vi "DroneTcpConnectionMovement.vi"() -> ()   [LabVIEW 2017]
uses:
  <vilib>/userdefined/High Color/IMAQdx.ctl
  <vilib>/vision/driver/IMAQdx.llb/IMAQdx Camera Control Mode.ctl
  <vilib>/vision/driver/NI_Vision_Acquisition_Software.lvlib
panel:
  in  "stop 3":bool
  in  "Snap":bool
  out "x":dbl
  out "created path":path
  in  "error in":errorcluster
  in  "Image Type":T1 items=["Grayscale (U8)", "Grayscale (I16)", "Grayscale (SGL)", "Complex (CSG)", "RGB (U32)", "HSL (U32)", "RGB (U64)", "Grayscale (U16)"]
  in  "Session In":T2
  in  "stop 2":bool
  out "Image":T3(plugin-control)
  out "unsigned byte array":u8[](array[numeric])
  out "Python server reply":string
  in  "stop":bool
  out "Control cluster":T4 {"Roll" scale=-1.0..1.0; "Pitch" scale=-1.0..1.0; "Vertical Speed" scale=-1.0..1.0; "Yaw Speed" scale=-1.0..1.0}
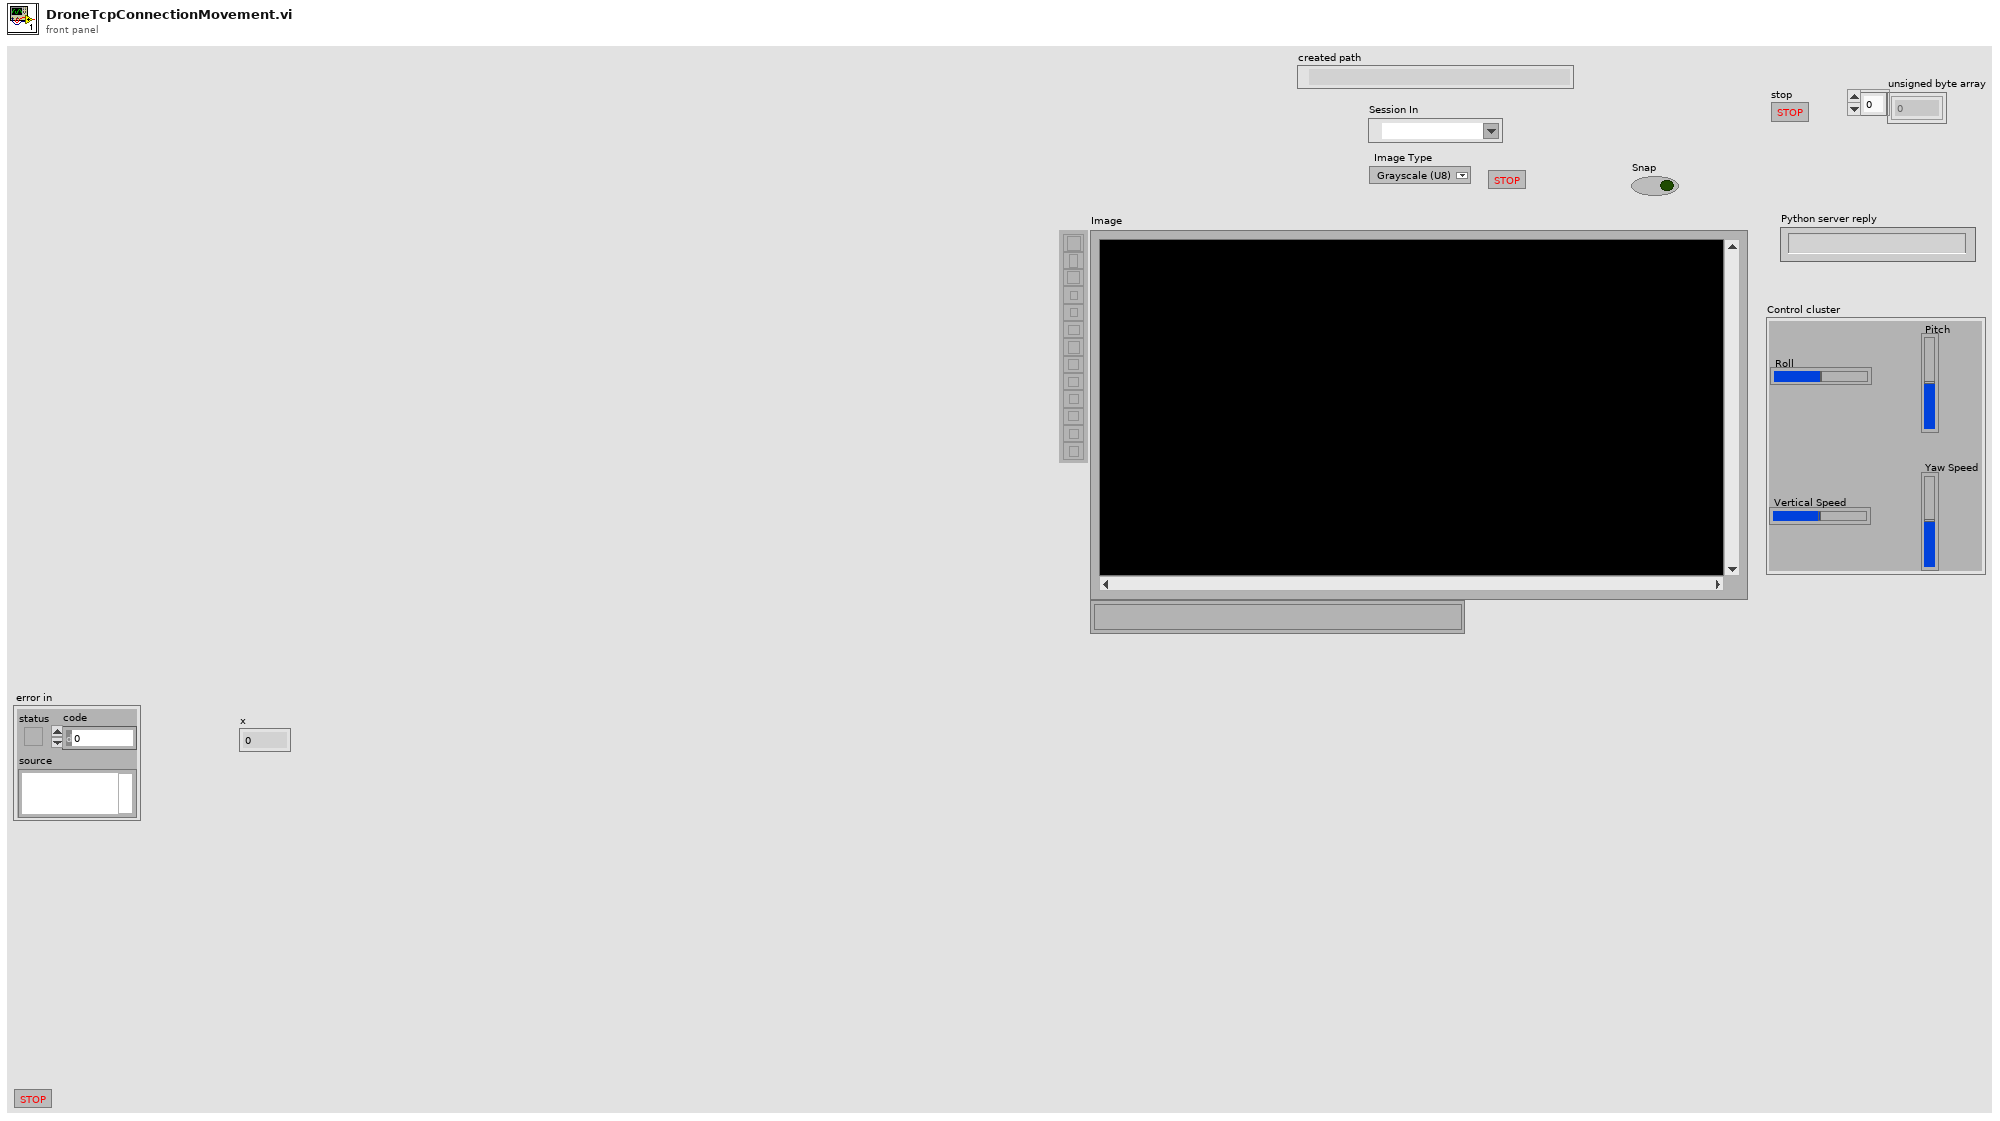
[diagram p1: front panel]
types:
  T1 = typedef "Image Type" = u32
  T2 = typedef "IMAQdx.ctl" = refnum<k21>
  T3 = typedef "IMAQ Image.ctl" = refnum<image>
  T4 = cluster{"Roll":dbl, "Pitch":dbl, "Vertical Speed":dbl, "Yaw Speed":dbl}
  T5 = typedef "NI_Vision_Acquisition_Software.lvlib/IMAQdx Camera Control Mode.ctl" = enum32{"Controller", "Listener"}
  T6 = cluster{"Boolean array[0]":bool, "Boolean array[1]":bool, "Boolean array[2]":bool, "Boolean array[3]":bool, "Boolean array[4]":bool, "Boolean array[5]":bool, "Boolean array[6]":bool, "Boolean array[7]":bool, "Boolean array[8]":bool}
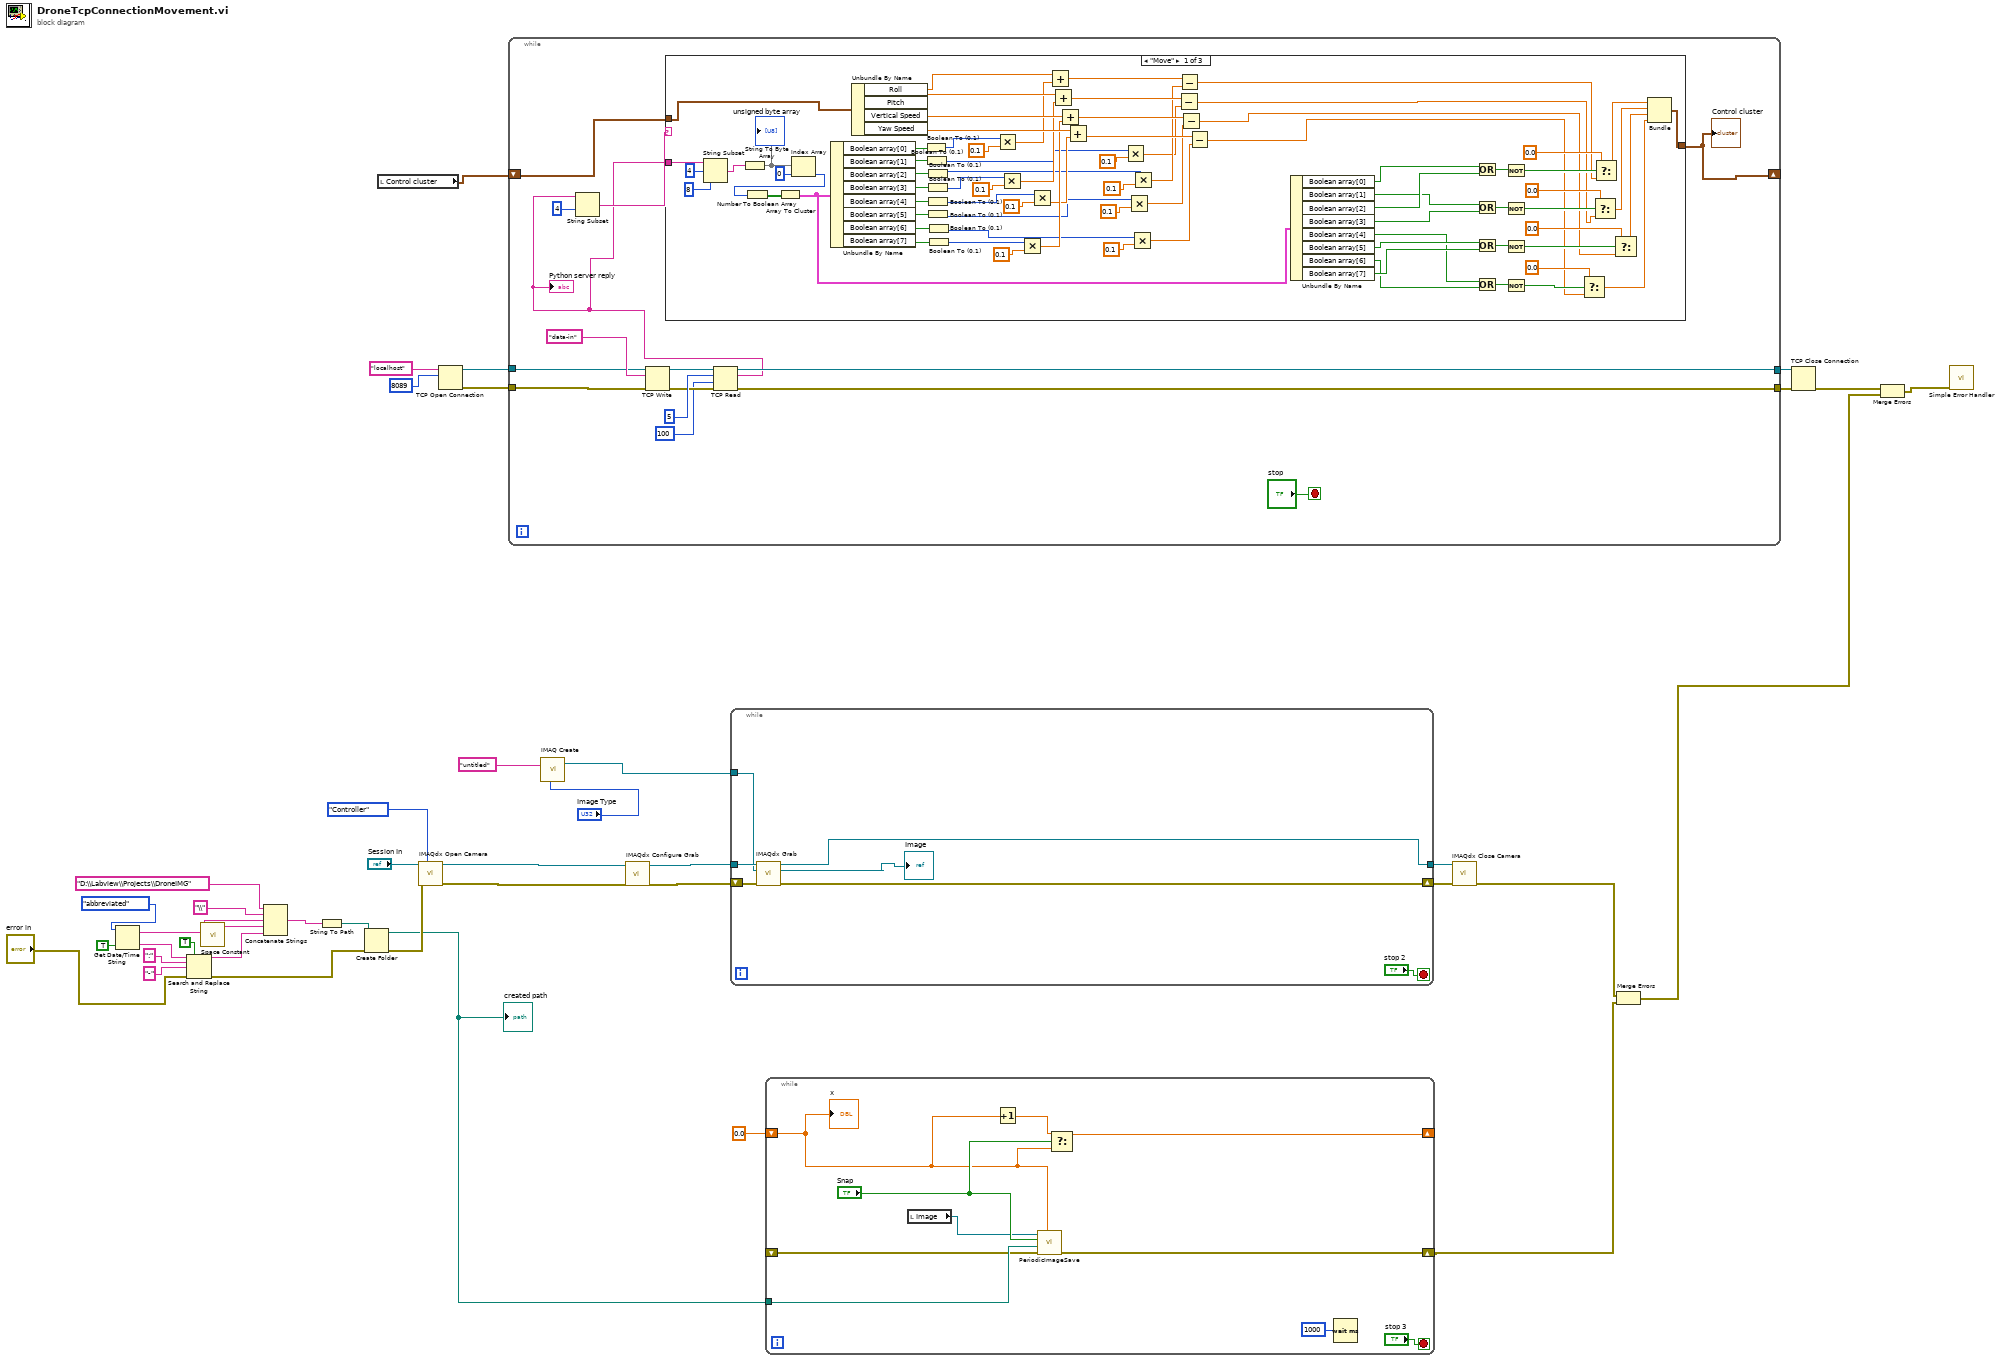
[diagram p0: block diagram]
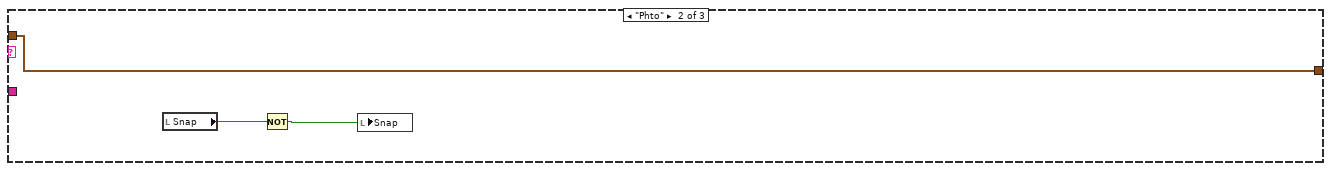
[diagram p2: hidden frame]
diagram:
  n1 = Get Date/Time String(date format (0)=enum16{"short", "long", "abbreviated"}."abbreviated", want seconds? (F)=TRUE) -> (date string=w26:string, time string=w23:string)  [unwired: 1 in]
  n2 = Search and Replace String(replace all?=TRUE ("replace all? (F)"), input string=w23, search string=":" ("replace string (\"\")"), replace string="-" ("replace string (\"\")"), error in="error in") -> (result string=w24:string, error out=w12:errorcluster)  [unwired: 3 in, 2 out]
  n3 = call <vilib>:"Space Constant.vi"() -> ("String"=w25:string)
  n4 = Concatenate Strings("D:\\Labview\\Projects\\DroneIMG" ("string"), "\\" ("string"), w26, w25, w24) -> (w15:string)
  n5 = String To Path(string=w15) -> (path=w14:path)
  n6 = Create Folder(path (use dialog)=w14, error in=w12) -> (created path=w10:path, error out=w11:errorcluster)  [unwired: 1 in, 1 out]
  "created path" <- w10
  n7 = local read "Control cluster"() -> (w36:T4)
  n8 = call <vilib>:"IMAQdx Open Camera.vi"("Camera Control Mode"=IMAQdx_Camera_Control_Mode."Controller", "error in"=w11, "Session In"="Session In") -> ("error out"=w3:errorcluster, "Session Out"=w31:T2)  [unwired: 7 in]
  n9 = TCP Open Connection(address="localhost", remote port or service name=u16 8089) -> (connection ID=w37:refnum<k5>, error out=w33:errorcluster)  [unwired: 3 in]
  n10 = while {
    tunnel: [w50] -> w41
    tunnel: [w49] -> w40
    tunnel: w33 -> [w42]
    tunnel: w37 -> [w48]
    shift-right: [w43] -> _
    shift-left: w36 -> [w45]
    stop <- "stop" stop-if-true
    n11 = TCP Write(connection ID=w48, data in="data-in", error in (no error)=w42) -> (connection ID out=w55:refnum<k5>, error out=w54:errorcluster)  [unwired: 1 in, 1 out]
    n12 = TCP Read(connection ID=w55, bytes to read=5, error in (no error)=w54, 9:100 ("timeout ms (25000)")) -> (connection ID out=w50:refnum<k5>, data out=w44:string, error out=w49:errorcluster)  [unwired: 1 in]
    "Python server reply" <- w44
    n13 = String Subset(string=w44, length (rest)=4 ("length (rest)")) -> (substring=w46:string)  [unwired: 1 in]
    n14 = case shown="\"Move\"" w46 {
      tunnel: [w128 w136 w139] -> w43
      tunnel: w45 -> [w129 w136 w139]
      tunnel: w44 -> [w135 _ _]
      frame "Move" {
        n15 = String Subset(string=w135, offset (0)=4, length (rest)=8 ("length (rest)")) -> (substring=w132:string)
        n16 = String To Byte Array(string=w132) -> (unsigned byte array=w131:u8[])
        "unsigned byte array" <- w131
        n17 = Index Array(array=w131, index=0) -> (element=w110:u8)
        n18 = Number To Boolean Array(number=w110) -> (Boolean array=w127:bool[])
        n19 = Array To Cluster(array=w127) -> (cluster=w73:T6)
        n20 = Unbundle By Name(w73) -> ("Boolean array[0]"=w118:bool, "Boolean array[1]"=w117:bool, "Boolean array[2]"=w116:bool, "Boolean array[3]"=w115:bool, "Boolean array[4]"=w114:bool, "Boolean array[5]"=w113:bool, "Boolean array[6]"=w112:bool, "Boolean array[7]"=w111:bool)
        n21 = Unbundle By Name(w129) -> ("Roll"=w126:dbl, "Pitch"=w124:dbl, "Vertical Speed"=w122:dbl, "Yaw Speed"=w120:dbl)
        n22 = Boolean To (0,1)(Boolean=w118) -> (0, 1=w98:i16)
        n23 = Boolean To (0,1)(Boolean=w117) -> (0, 1=w87:i16)
        n24 = Boolean To (0,1)(Boolean=w116) -> (0, 1=w89:i16)
        n25 = Boolean To (0,1)(Boolean=w115) -> (0, 1=w102:i16)
        n26 = Boolean To (0,1)(Boolean=w114) -> (0, 1=w101:i16)
        n27 = Boolean To (0,1)(Boolean=w113) -> (0, 1=w93:i16)
        n28 = Boolean To (0,1)(Boolean=w112) -> (0, 1=w96:i16)
        n29 = Boolean To (0,1)(Boolean=w111) -> (0, 1=w108:i16)
        n30 = Multiply(x=w98, y=0.1) -> (x*y=w99:dbl)
        n31 = Multiply(x=w102, y=0.1) -> (x*y=w103:dbl)
        n32 = Multiply(x=w108, y=0.1) -> (x*y=w107:dbl)
        n33 = Multiply(x=w101, y=0.1) -> (x*y=w105:dbl)
        n34 = Add(x=w126, y=w99) -> (x+y=w125:dbl)
        n35 = Add(x=w124, y=w103) -> (x+y=w123:dbl)
        n36 = Add(x=w122, y=w107) -> (x+y=w121:dbl)
        n37 = Add(x=w120, y=w105) -> (x+y=w119:dbl)
        n38 = Multiply(x=w87, y=0.1) -> (x*y=w86:dbl)
        n39 = Multiply(x=w93, y=0.1) -> (x*y=w92:dbl)
        n40 = Multiply(x=w96, y=0.1) -> (x*y=w95:dbl)
        n41 = Multiply(x=w89, y=0.1) -> (x*y=w88:dbl)
        n42 = Subtract(x=w123, y=w86) -> (x-y=w60:dbl)
        n43 = Subtract(x=w125, y=w88) -> (x-y=w58:dbl)
        n44 = Subtract(x=w121, y=w92) -> (x-y=w62:dbl)
        n45 = Subtract(x=w119, y=w95) -> (x-y=w64:dbl)
        n46 = Unbundle By Name(w73) -> ("Boolean array[0]"=w72:bool, "Boolean array[1]"=w70:bool, "Boolean array[2]"=w71:bool, "Boolean array[3]"=w69:bool, "Boolean array[4]"=w66:bool, "Boolean array[5]"=w67:bool, "Boolean array[6]"=w65:bool, "Boolean array[7]"=w68:bool)
        n47 = Or(x=w72, y=w71) -> (x .or. y?=w85:bool)
        n48 = Or(x=w70, y=w69) -> (x .or. y?=w82:bool)
        n49 = Or(x=w67, y=w68) -> (x .or. y?=w79:bool)
        n50 = Or(x=w66, y=w65) -> (x .or. y?=w76:bool)
        n51 = Not(x=w85) -> (.not. x?=w84:bool)
        n52 = Not(x=w82) -> (.not. x?=w81:bool)
        n53 = Not(x=w79) -> (.not. x?=w78:bool)
        n54 = Not(x=w76) -> (.not. x?=w75:bool)
        n55 = Select(t=0.0, s=w75, f=w64) -> (s? t:f=w63:dbl)
        n56 = Select(t=0.0, s=w81, f=w60) -> (s? t:f=w59:dbl)
        n57 = Select(t=0.0, s=w84, f=w58) -> (s? t:f=w57:dbl)
        n58 = Select(t=0.0, s=w78, f=w62) -> (s? t:f=w61:dbl)
        n59 = Bundle("t"=w57, "t"=w59, "t"=w61, "t"=w63) -> (w128:cluster{"t":dbl, "t":dbl, "t":dbl, "t":dbl})  [unwired: 1 in]
      }
      frame "Phto" {
        n60 = local read "Snap"() -> (w138:bool)
        n61 = Not(x=w138) -> (.not. x?=w137:bool)
        n62 = local write "Snap"(w137) -> ()
      }
      frame " ", Default {
      }
    }
    "Control cluster" <- w43
  }
  n63 = call "IMAQ Create"("Image Name"="untitled", "Image Type"="Image Type") -> ("New Image"=w6:T3)  [unwired: 3 in, 1 out]
  n64 = call <vilib>:"IMAQdx Configure Grab.vi"("error in"=w3, "Session In"=w31) -> ("error out"=w2:errorcluster, "Session Out"=w30:T2)  [unwired: 8 in]
  n65 = while {
    tunnel: w30 -> [w145]
    tunnel: [w143] -> w27
    shift-right: [w141] -> w8
    shift-left: w2 -> [w144]
    tunnel: w6 -> [w142]
    stop <- "stop 2" stop-if-true
    n66 = call <vilib>:"IMAQdx Grab.vi"("error in"=w144, "Image In"=w142, "Session In"=w145) -> ("error out"=w141:errorcluster, "Image Out"=→"Image":T3, "Session Out"=w143:T2)  [unwired: 5 in, 1 out]
  }
  n67 = while {
    shift-right: [w150] -> _
    shift-left: 0.0 -> [w151]
    tunnel: w10 -> [w154]
    shift-right: [w147] -> w7
    shift-left: _ -> [w148]
    stop <- "stop 3" stop-if-true
    n68 = local read "Image"() -> (w149:T3)
    n69 = Increment(x=w151) -> (x+1=w152:dbl)
    n70 = call "PeriodicImageSave.vi"("x"=w151, "error in (no error)"=w148, "in path"=w154, "Snap"="Snap", "Image In"=w149) -> ("error out"=w147:errorcluster)  [unwired: 5 in]
    n71 = Select(t=w152, s="Snap", f=w151) -> (s? t:f=w150:dbl)
    n72 = Wait (ms)(milliseconds to wait=u32 1000) -> ()  [unwired: 1 out]
    "x" <- w151
  }
  n73 = call <vilib>:"IMAQdx Close Camera.vi"("error in"=w8, "Session In"=w27) -> ("error out"=w5:errorcluster)  [unwired: 9 in]
  n74 = Merge Errors(w5, w7) -> (w1:errorcluster)
  n75 = TCP Close Connection(connection ID=w41, error in (no error)=w40) -> (error out=w35:errorcluster)  [unwired: 1 in, 1 out]
  n76 = Merge Errors(w35, w1) -> (w34:errorcluster)
  n77 = call <vilib>:"Simple Error Handler.vi"("error in (no error)"=w34) -> ()  [unwired: 4 in, 5 out]
